vi "Global_CMD to SM Data.vi"() -> ()   [LabVIEW 2017, in "MechamunDrive.lvlib"]
uses:
  MechamunDrive.lvlib
  Cluster_CMD to SM Data.ctl
  Enum_SM Cmd Select.ctl
panel:
  in  "CMD Drive Data":T1
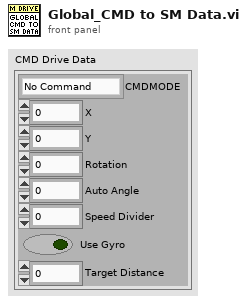
[diagram p1: front panel]
types:
  T1 = typedef "MechamunDrive.lvlib/Cluster_CMD to SM Data.ctl" = cluster{"CMDMODE":T2, "X":dbl, "Y":dbl, "Rotation":dbl, "Auto Angle":dbl, "Speed Divider":dbl, "Use Gyro":bool, "Target Distance":dbl}
  T2 = typedef "MechamunDrive.lvlib/Enum_SM Cmd Select.ctl" = enum16{"No Command", "Halt", "Manual Keep Rotation", "Manual", "Track Front", "Track Rotation", "Track Lateral", "Track Vision Lat", "Track Vision Rot", "Strafe Right", "Strafe Left"}
diagram:
